vi "CALC_Conditions_and_agreement.vi"(8 "error in (no error)":T1, 9 "Reset? (F)":bool, 10 "Array of conditions":T2 {"Response"."TTL pulse length, ms" min=0.0 max=10000.0 step=10.0 format="%0.0g"; "Specifier(s)"."Validity criteria(s)"."Validity value" min=0.0 step=0.1 format="%.2g"; "Specifier(s)"."Value" step=1.0 format="%#.2g"}, 11 "Data frame in":T7) -> (0 "error out":T1, 3 "Activated conditions":bool[](array[boolean]))   [LabVIEW 2018, in "Tracker.lvlib"]
uses:
  Tracker.lvlib
  Controls/CTL_Animal_Coordinates_and_Speed.ctl
  Controls/CTL_Full_data_frame.ctl
  Controls/CTL_Conditions_Cluster.ctl
  Controls/CTL_Condition_type.ctl
  Controls/CTL_Comparison_type.ctl
  Controls/CTL_Validity_check_criteria.ctl
  Controls/CTL_Condition_response_type.ctl
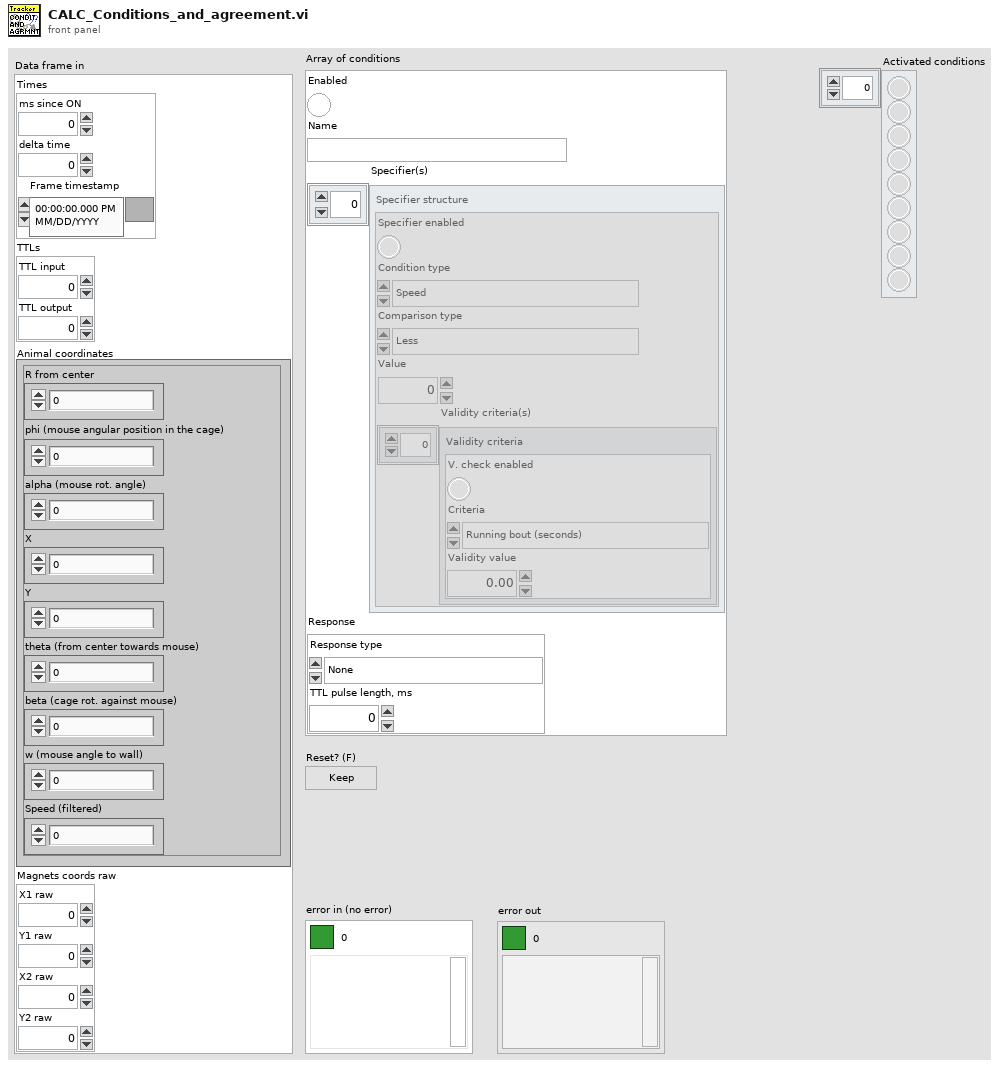
[diagram p1: front panel]
types:
  T1 = cluster{"Boolean Round":bool, "code":i32, "source":string}
  T2 = typedef "Tracker.lvlib/CTL_Conditions_Cluster.ctl" = cluster{"Enabled":bool, "Name":string, "Specifier(s)":cluster{"Specifier enabled":bool, "Condition type":T3, "Limit type":T4, "Value":dbl, "Validity criteria(s)":cluster{"V. check enabled":bool, "Criteria":T5, "Validity value":dbl}[]}[], "Response":cluster{"Response type":T6, "TTL pulse length, ms":dbl}}
  T3 = typedef "Tracker.lvlib/CTL_Condition_type.ctl" = enum16{"Not in use", "Speed", "Zone", "Angle to wall"}
  T4 = typedef "Tracker.lvlib/CTL_Comparison_type.ctl" = enum16{"Less", "Less or Equal", "Equal", "Greater or Equal", "Greater", "Not Equal"}
  T5 = typedef "Tracker.lvlib/CTL_Validity_check_criteria.ctl" = enum16{"Running bout (seconds)", "Running bout (meters)"}
  T6 = typedef "Tracker.lvlib/CTL_Condition_response_type.ctl" = enum16{"None", "TTL"}
  T7 = typedef "Tracker.lvlib/CTL_Full_data_frame.ctl" = cluster{"Times":cluster{"ms since ON":u32, "delta time":u32, "Frame timestamp":timestamp}, "TTLs":cluster{"TTL input":i16, "TTL output":i16}, "Animal coordinates":T8, "Magnets coords raw":cluster{"X1 raw":dbl, "Y1 raw":dbl, "X2 raw":dbl, "Y2 raw":dbl}}
  T8 = typedef "Tracker.lvlib/CTL_Animal_Coordinates_and_Speed.ctl" = cluster{"R from center":dbl, "phi (mouse angular position in the cage)":dbl, "alpha (mouse rot. angle)":dbl, "X":dbl, "Y":dbl, "theta (from center towards mouse)":dbl, "beta (cage rot. against mouse)":dbl, "w (mouse angle to wall)":dbl, "Speed (filtered)":dbl}
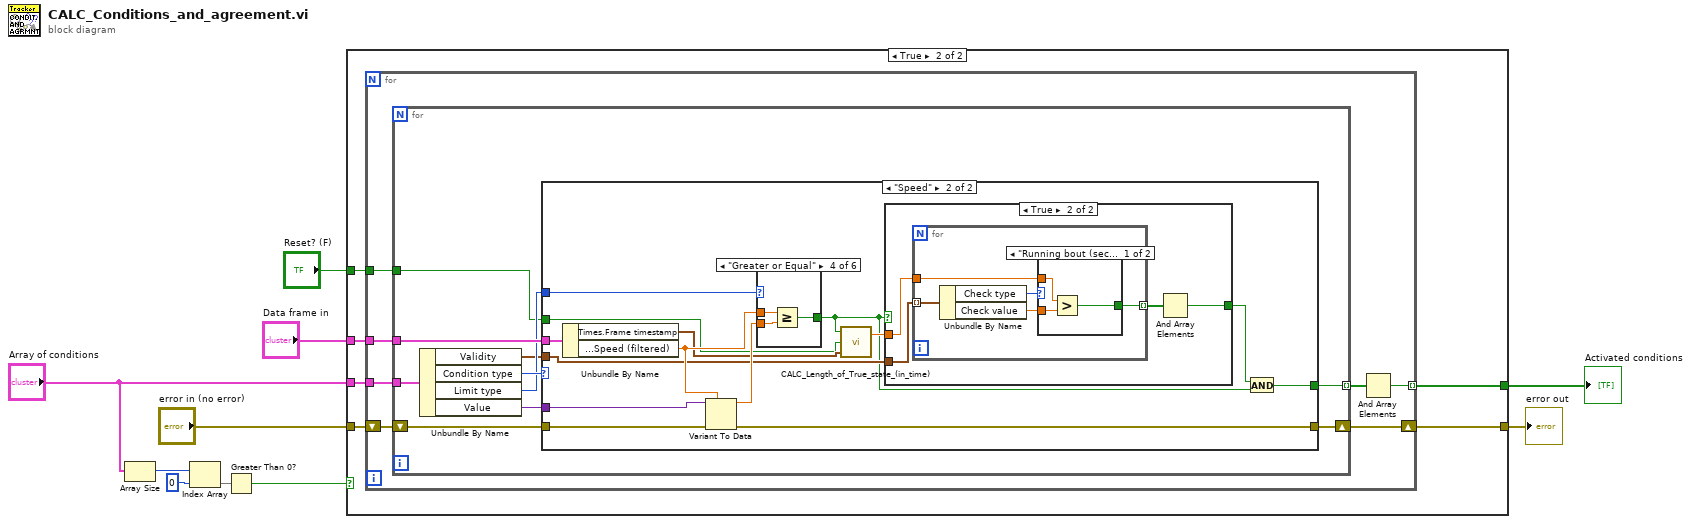
[diagram p0: block diagram]
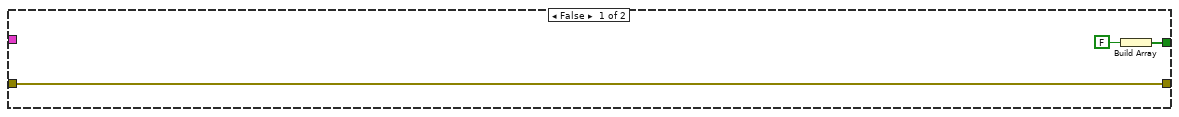
[diagram p2: hidden frame]
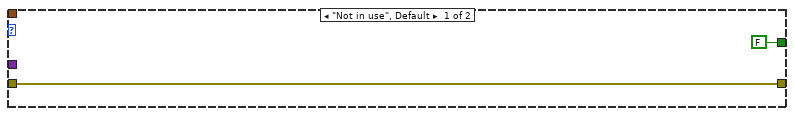
[diagram p3: hidden frame]
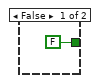
[diagram p4: hidden frame]
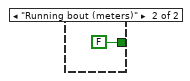
[diagram p5: hidden frame]
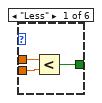
[diagram p6: hidden frame]
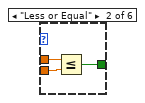
[diagram p7: hidden frame]
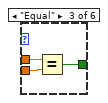
[diagram p8: hidden frame]
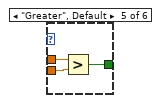
[diagram p9: hidden frame]
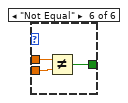
[diagram p10: hidden frame]
diagram:
  n1 = Array Size(array="Array of conditions") -> (size(s)=w4:i32)
  n2 = Index Array(array=w4, index=0) -> (element=w2)
  n3 = Greater Than 0?(x=w2) -> (x > 0?=w1:bool)
  n4 = case shown="True" w1 {
    tunnel: "Array of conditions" -> [_ w19]
    tunnel: "Data frame in" -> [_ w18]
    tunnel: "error in (no error)" -> [w11 w17]
    tunnel: [w11 w16] -> w8
    tunnel: [w12 w15] -> w7
    tunnel: "Reset? (F)" -> [_ w14]
    frame False {
      n5 = Build Array(FALSE) -> (w12:bool[])
    }
    frame True {
      n6 = for {
        tunnel: w19 -> [w26]
        tunnel: w18 -> [w25]
        shift-right: [w23] -> w16
        shift-left: w17 -> [w24]
        tunnel: [w21] -> w15 mode=indexing
        tunnel: w14 -> [w20]
        n7 = for {
          tunnel: w26 -> [w36]
          tunnel: w25 -> [w34]
          shift-right: [w30] -> w23
          shift-left: w24 -> [w31]
          tunnel: [w29] -> w22 mode=indexing
          tunnel: w20 -> [w28]
          n8 = Unbundle By Name(w36) -> ("Validity"=w27:cluster{"Check type":T5, "Check value":dbl}[], "Condition type"=w35:T3, "Limit type"=w33:T4, "Value"=w32:variant)
          n9 = case shown="\"Speed\"" w35 {
            tunnel: w34 -> [_ w52]
            tunnel: w33 -> [_ w50]
            tunnel: w32 -> [_ w51]
            tunnel: [FALSE w41] -> w29
            tunnel: w31 -> [w38 w47]
            tunnel: [w38 w46] -> w30
            tunnel: w28 -> [_ w44]
            tunnel: w27 -> [_ w43]
            frame "Not in use", Default {
            }
            frame "Speed" {
              n10 = Unbundle By Name(w52) -> ("Times.Frame timestamp"=w45:timestamp, "Animal coordinates.Speed (filtered)"=w48:dbl)
              n11 = Variant To Data(error in=w47, type=w48, Variant=w51) -> (data=w49:dbl, error out=w46:errorcluster)
              n12 = case shown="\"Greater or Equal\"" w50 {
                tunnel: w49 -> [w69 w72 w75 w78 w81 w84]
                tunnel: w48 -> [w68 w71 w74 w77 w80 w83]
                tunnel: [w67 w70 w73 w76 w79 w82] -> w39
                frame "Less" {
                  n13 = Less?(x=w68, y=w69) -> (x < y?=w67:bool)
                }
                frame "Less or Equal" {
                  n14 = Less Or Equal?(x=w71, y=w72) -> (x <= y?=w70:bool)
                }
                frame "Equal" {
                  n15 = Equal?(x=w74, y=w75) -> (x = y?=w73:bool)
                }
                frame "Greater or Equal" {
                  n16 = Greater Or Equal?(x=w77, y=w78) -> (x >= y?=w76:bool)
                }
                frame "Greater", Default {
                  n17 = Greater?(x=w80, y=w81) -> (0:w79:bool)
                }
                frame "Not Equal" {
                  n18 = Not Equal?(x=w83, y=w84) -> (x != y?=w82:bool)
                }
              }
              n19 = call "CALC_Length_of_True_state_(in_time).vi"("Frame timestamp"=w45, "Reset? (F)"=w44, "True state input"=w39) -> ("True was kept for, s"=w42:dbl)  [unwired: 1 in]
              n20 = case shown="True" w39 {
                tunnel: w43 -> [_ w57]
                tunnel: w42 -> [_ w56]
                tunnel: [FALSE w54] -> w40
                frame False {
                }
                frame True {
                  n21 = for {
                    tunnel: w57 -> [w62] mode=indexing
                    tunnel: w56 -> [w60]
                    tunnel: [w58] -> w55 mode=indexing
                    n22 = Unbundle By Name(w62) -> ("Check type"=w61:T5, "Check value"=w59:dbl)
                    n23 = case shown="\"Running bout (seconds)\", Default" w61 {
                      tunnel: w60 -> [w64 _]
                      tunnel: w59 -> [w65 _]
                      tunnel: [w63 FALSE] -> w58
                      frame "Running bout (seconds)", Default {
                        n24 = Greater?(x=w64, y=w65) -> (0:w63:bool)
                      }
                      frame "Running bout (meters)" {
                      }
                    }
                  }
                  n25 = And Array Elements(Boolean array=w55) -> (logical AND=w54:bool)
                }
              }
              n26 = And(x=w40, y=w39) -> (x .and. y?=w41:bool)
            }
          }
        }
        n27 = And Array Elements(Boolean array=w22) -> (logical AND=w21:bool)
      }
    }
  }
  "error out" <- w8
  "Activated conditions" <- w7
